vi "FTP Put and Get Files.vi"() -> ()   [LabVIEW 2023]
doc: "Demonstrates the use of the FTP VIs to \"put\" a binary file on an FTP server and \"get\" a text file from an FTP server."
uses:
  <vilib>/FTP/NI_FTP.lvlib
panel:
  out "Text in Retrieved File":string
  out "Retrieved File":path
  out "Sent File":path
  out "Data in Local File":dbl[](graph)
  # "Overview: Demonstrates the use of the FTP VIs to \"put\" a binary file on an FTP server and \"get\" a text file from an FTP server.\nInstructions:\nRun the VI."
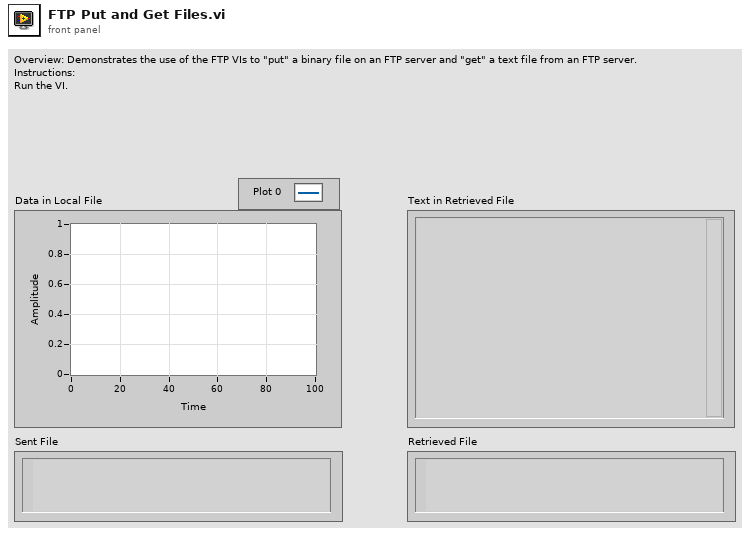
[diagram p1: front panel]
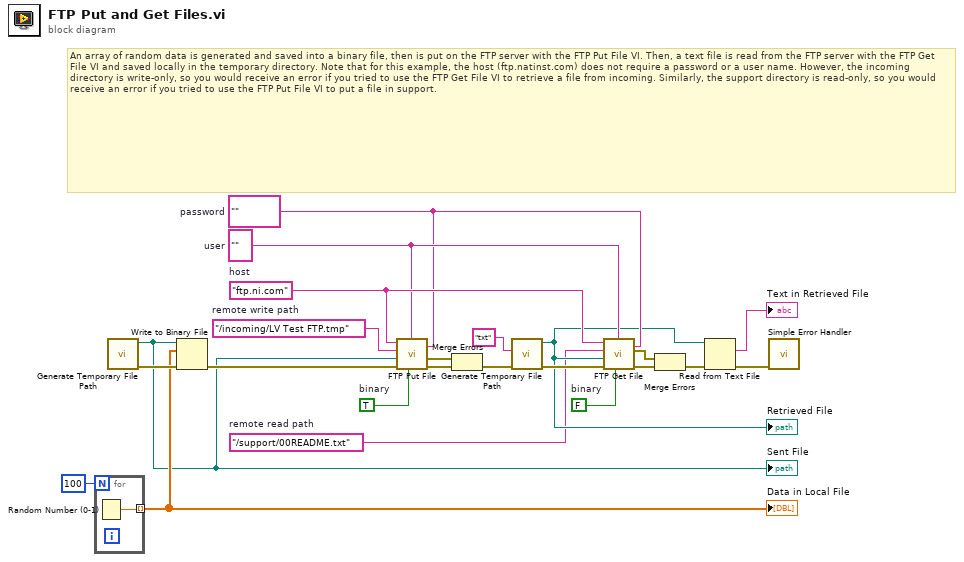
[diagram p0: block diagram]
diagram:
  w5 = FALSE  # binary
  w4 = "/support/00README.txt"  # remote read path
  w7 = ""  # password
  w8 = ""  # user
  w14 = TRUE  # binary
  w15 = "/incoming/LV Test FTP.tmp"  # remote write path
  w16 = "ftp.ni.com"  # host
  # "An array of random data is generated and saved into a binary file, then is put on the FTP server with the FTP Put File VI. Then, a text file is read from the FTP server with the FTP Get File VI and saved locally in the temporary directory. Note that for this example, the host (ftp.natinst.com) does not require a password or a user name. However, the incoming directory is write-only, so you would receive an error if you tried to use the FTP Get File VI to retrieve a file from incoming. Similarly, the support directory is read-only, so you would receive an error if you tried to use the FTP Put File VI to put a file in support."
  n1 = for {
    N: 100 -> [_]
    tunnel: [w24] -> w21 mode=indexing
    n2 = Random Number (0-1)() -> (number: 0 to 1=w24:dbl)
  }
  "Data in Local File" <- w21
  n3 = call <vilib>:"Generate Temporary File Path.vi"() -> ("error out"=w22:errorcluster, "Unique Temporary File Path"=w1:path)  [unwired: 10 in]
  "Sent File" <- w1
  n4 = Write to Binary File(file (use dialog)=w1, data=w21, error in=w22) -> (error out=w20:errorcluster)  [unwired: 3 in, 2 out]
  n5 = call <vilib>:"FTP Put File.vi"("password"=w7, "binary (F)"=w14, "user"=w8, "error in (no error)"=w20, "local path"=w1, "remote path"=w15, "host"=w16) -> ("error out"=w19:errorcluster, "file error"=w17:errorcluster)  [unwired: 3 in]
  n6 = Merge Errors(w17, w19) -> (w18:errorcluster)
  n7 = call <vilib>:"Generate Temporary File Path.vi"("error in (no error)"=w18, "Temporary File Extension (tmp)"="txt") -> ("error out"=w13:errorcluster, "Unique Temporary File Path"=w6:path)  [unwired: 8 in]
  "Retrieved File" <- w6
  n8 = call <vilib>:"FTP Get File.vi"("password"=w7, "binary (F)"=w5, "user"=w8, "error in (no error)"=w13, "local path"=w6, "remote path"=w4, "host"=w16) -> ("error out"=w12:errorcluster, "file error"=w11:errorcluster)  [unwired: 3 in]
  n9 = Merge Errors(w11, w12) -> (w10:errorcluster)
  n10 = Read from Text File(file (use dialog)=w6, error in=w10) -> (text=→"Text in Retrieved File":string, error out=w9:errorcluster)  [unwired: 2 in, 2 out]
  n11 = call <vilib>:"Simple Error Handler.vi"("error in (no error)"=w9) -> ()  [unwired: 4 in, 5 out]
